vi "DCS.vi"(3 "error in":errorcluster) -> (10 "error out":errorcluster)   [LabVIEW 2012]
uses:
  Database2.0/Private/dcs points.ctl
  Database2.0/Private/dcs_spot.ctl
  <vilib>/DAQmx/read.llb/DAQmx Read (Analog 1D Wfm NChan NSamp).vi
  <vilib>/DAQmx/create/channels.llb/DAQmx Create Channel (AI-Voltage-Basic).vi
  <vilib>/DAQmx/configure/timing.llb/DAQmx Timing (Sample Clock).vi
  <vilib>/DAQmx/configure/trigger.llb/DAQmx Reference Trigger (Digital Edge).vi
  <vilib>/DAQmx/miscellaneous.llb/DAQmx Fill In Error Info.vi
  <vilib>/gmath/NumericalOptimization/Nonlinear Curve Fit LM.vi
  <vilib>/gmath/NI_Gmath.lvlib
panel:
  in  "Color bar Control":cluster{dbl, u32}[](array[cluster])
  in  "stop":bool
  in  "Tab Control":T1(tab)
  out "Intensity Graph":dbl[][](graph)
  in  "Spot Save Folder":path=path "C:/Users/Clavius/Desktop/Spot Images"
  in  "Save Spot Image":bool
  in  "Clear Spot/Track":bool
  in  "Particle Limit":i64=500 min=0 step=10
  out "Laser spot\nMove (mm)":dbl[](array[numeric])=[nan, nan] format="%#.3g"
  out "Avg. Freq. (Hz)":dbl
  in  "Orange Cursor Position":dbl[](array[numeric])=[0.0, 0.0] min=-12.0 max=12.0 step=0.1 format="%.3g"
  out "Spot Widths":dbl[](array[numeric]) format="%.6g"
  out "Countdown to\nnext track point":i32=1
  out "XY Graph":cluster{"Y":dbl[], "Y":dbl[]}[](graph)
  in  "Load old position\nto Orange Cursor":bool
  in  "Set Orange Cursor\nto current position":bool
  out "# of Particles\nin Spot":dbl
  out "Current Spot Pos":dbl[](array[numeric])=[nan, nan] format="%.3g"
  in  "# of shots to calculate spot":i32=20
  out "Spot Size over time":dbl[][](graph)
  out "Detector/trigger":waveform(dbl)[](graph)=[{"t0"=timestamp(3437998856.7399178 s since 1904-01-01), "dt"=4.999999999999997e-05, "Y"=[]}] caption="Measurement"
  out "Top to Bottom":waveform(dbl)[](graph)=[{"t0"=timestamp(0 s since 1904-01-01), "dt"=4.999999999999997e-05, "Y"=[]}, {"t0"=timestamp(0 s since 1904-01-01), "dt"=4.999999999999997e-05, "Y"=[]}, {"t0"=timestamp(0 s since 1904-01-01), "dt"=4.999999999999997e-05, "Y"=[]}, {"t0"=timestamp(0 s since 1904-01-01), "dt"=4.999999999999997e-05, "Y"=[]}] caption="Measurement"
  out "Left to Right":waveform(dbl)[](graph)=[{"t0"=timestamp(0 s since 1904-01-01), "dt"=4.999999999999997e-05, "Y"=[]}, {"t0"=timestamp(0 s since 1904-01-01), "dt"=4.999999999999997e-05, "Y"=[]}, {"t0"=timestamp(0 s since 1904-01-01), "dt"=4.999999999999997e-05, "Y"=[]}, {"t0"=timestamp(0 s since 1904-01-01), "dt"=4.999999999999997e-05, "Y"=[]}] caption="Measurement"
  out "All Signals":waveform(dbl)[](graph)=[{"t0"=timestamp(3437998856.7398734 s since 1904-01-01), "dt"=4.999999999999997e-05, "Y"=[]}, {"t0"=timestamp(3437998856.739879 s since 1904-01-01), "dt"=4.999999999999997e-05, "Y"=[]}, {"t0"=timestamp(3437998856.7398844 s since 1904-01-01), "dt"=4.999999999999997e-05, "Y"=[]}, {"t0"=timestamp(3437998856.73989 s since 1904-01-01), "dt"=4.999999999999997e-05, "Y"=[]}, {"t0"=timestamp(3437998856.739896 s since 1904-01-01), "dt"=4.999999999999997e-05, "Y"=[]}, {"t0"=timestamp(3437998856.739901 s since 1904-01-01), "dt"=4.999999999999997e-05, "Y"=[]}, {"t0"=timestamp(3437998856.739907 s since 1904-01-01), "dt"=4.999999999999997e-05, "Y"=[]}, {"t0"=timestamp(3437998856.7399125 s since 1904-01-01), "dt"=4.999999999999997e-05, "Y"=[]}, {"t0"=timestamp(3437998856.7399178 s since 1904-01-01), "dt"=4.999999999999997e-05, "Y"=[]}] caption="Measurement"
  in  "timeout":dbl=2.0 format="%0.2f"
  out "Running Errors":errorcluster
  in  "source":tag="/Dev6/PFI0"
  in  "Detector":tag="Dev6/ai8"
  in  "B2":tag="Dev6/ai4" caption="B2 /6"
  in  "B1":tag="Dev6/ai5" caption="B1 /5"
  in  "T1":tag="Dev6/ai6" caption="T1 /8"
  in  "T2":tag="Dev6/ai7" caption="T2 /7"
  in  "R2":tag="Dev6/ai3" caption="R2 /3"
  in  "R1":tag="Dev6/ai2" caption="R1 /4"
  in  "L1":tag="Dev6/ai1" caption="L1 /1"
  in  "pretrigger samples per channel":u32=120
  in  "slope":i32(ring)=10280 items=["Rising"=10280, "Falling"=10171]
  in  "Maximum Value":dbl=10.0 format="%0.2f"
  in  "Minimum Value":dbl=-10.0 format="%0.2f"
  in  "Rate":dbl=20000.0 caption="Sample Rate (Hz)" format="%0.2f"
  in  "Samples per Channel":i32=500
  in  "L2":tag="Dev6/ai0" caption="L2 /2"
  in  "Clear DCS errors":bool
  # "Channel Parameters"
  # "Timing Parameters"
  # "Trigger Parameters"
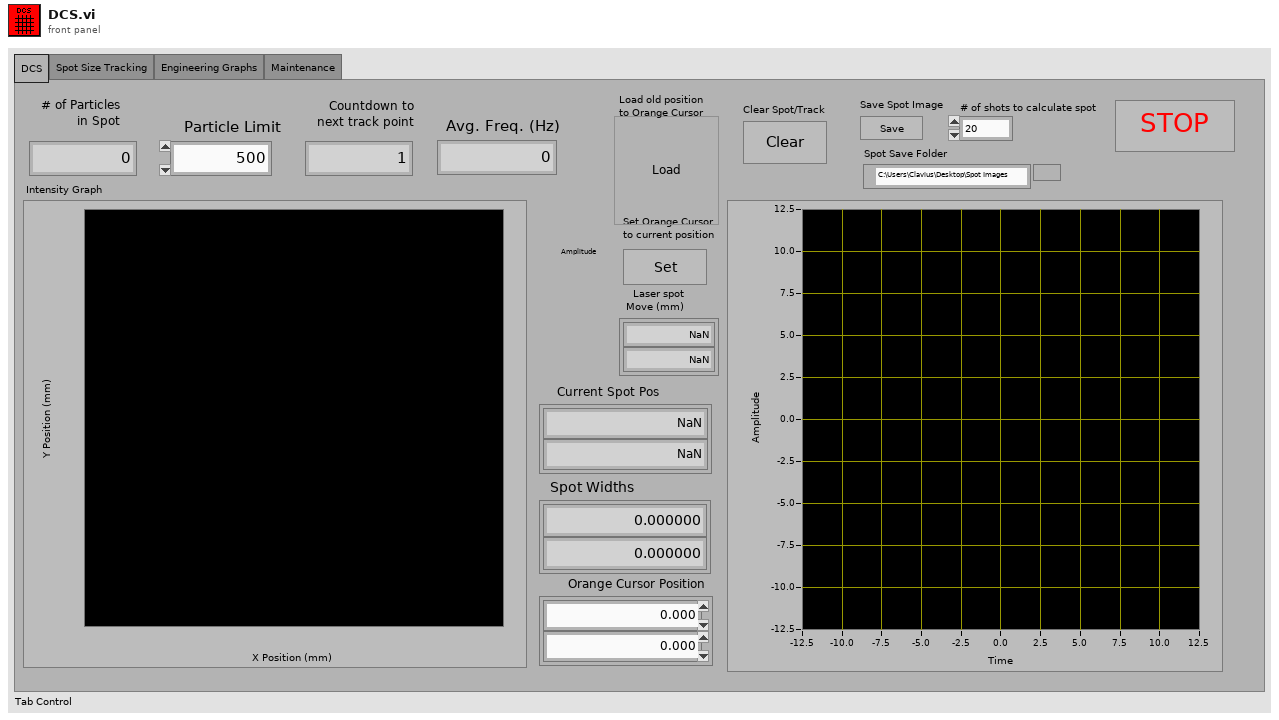
[diagram p1: front panel]
types:
  T1 = enum32{"DCS", "Spot Size Tracking", "Engineering Graphs", "Maintenance"}
  T2 = typedef "dcs_spot.ctl" = cluster{"DCS spot ID":i32, "Integer Timestamp":i64, "Spot X":dbl, "Spot Y":dbl, "Spot Width X":dbl, "Spot Width Y":dbl, "Spot Size":i32, "Experiment Settings ID":i32}
  T3 = typedef "dcs points.ctl" = cluster{"Integer Timestamp":i64, "X":dbl, "Y":dbl, "DCS spot ID":i32}
  T4 = typedef "imagedata.ctl" = cluster{"image type":i32, "image depth":i32, "image":u8[], "mask":u8[], "colors":u32[], "Rectangle":cluster{"left":i16, "top":i16, "right":i16, "bottom":i16}}
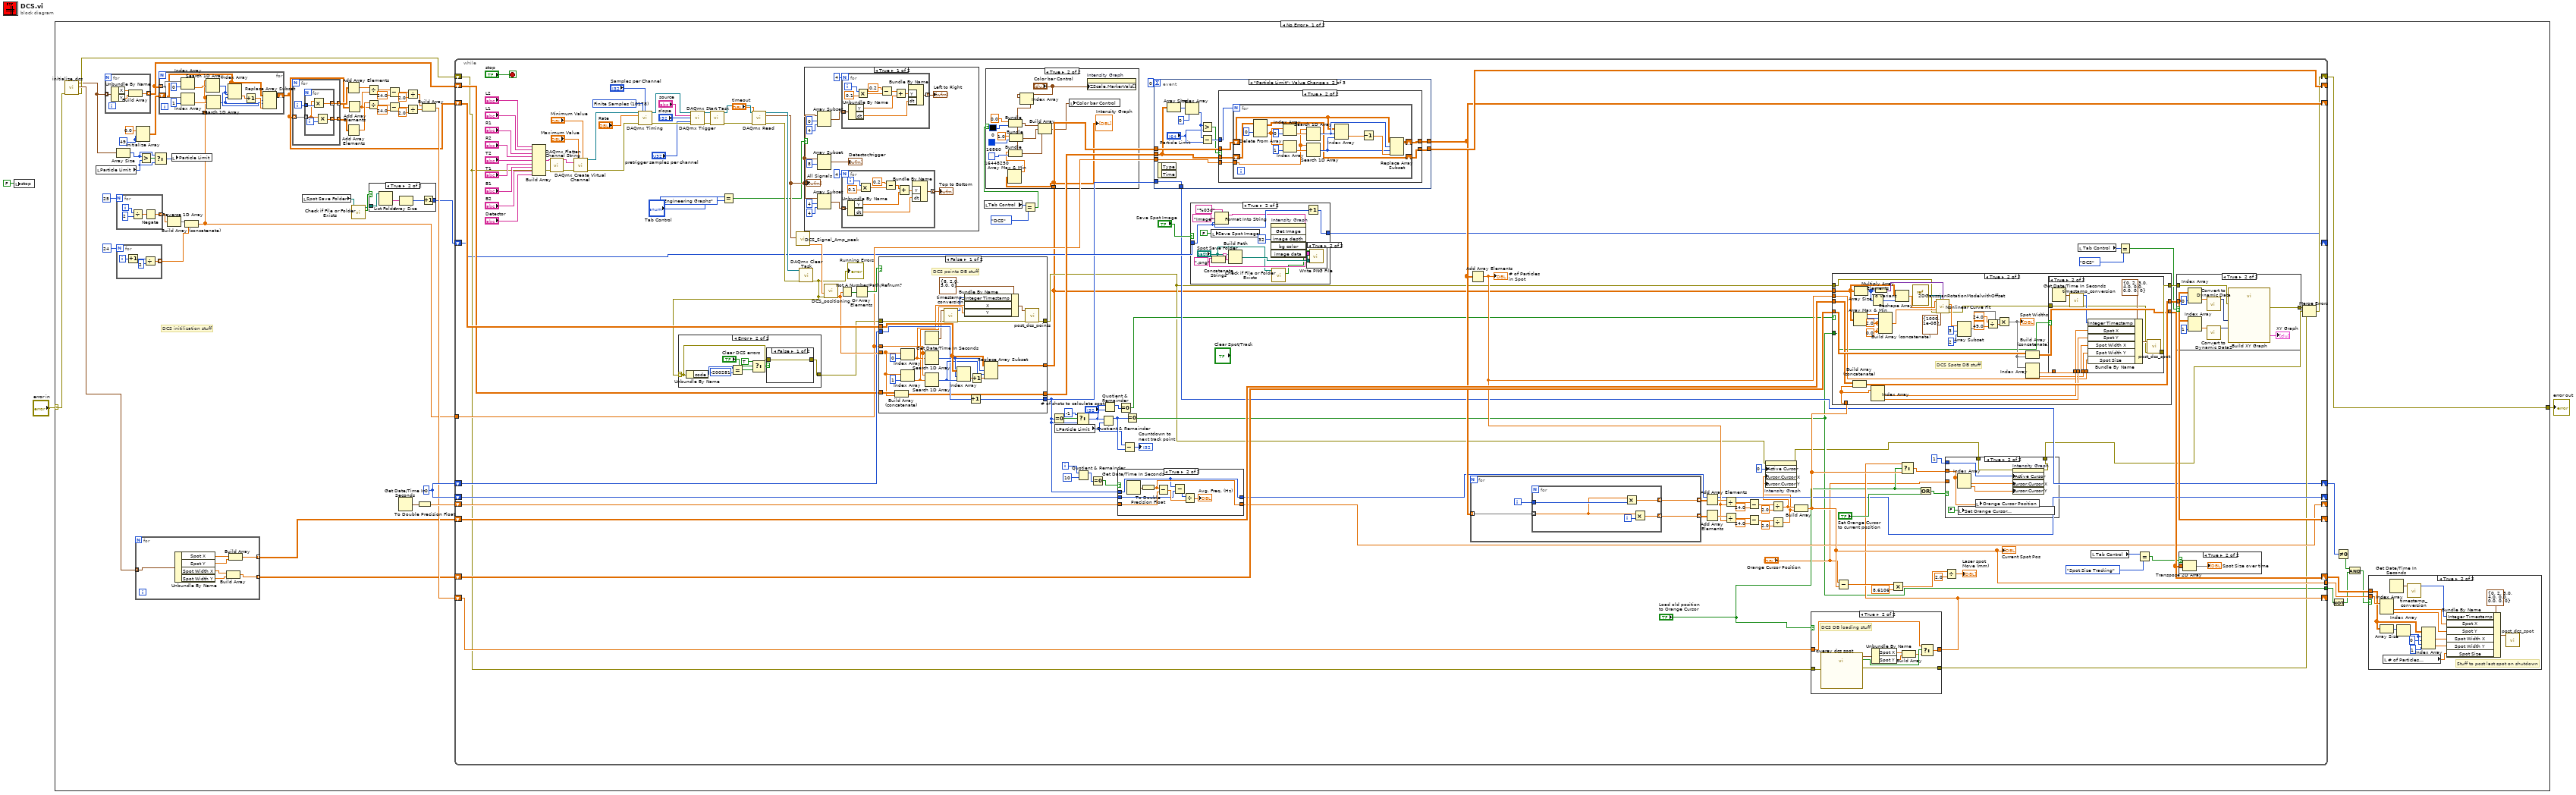
[diagram p0: block diagram]
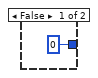
[diagram p2: hidden frame]
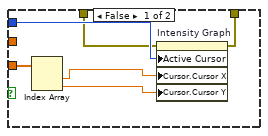
[diagram p7: hidden frame]
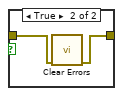
[diagram p12: hidden frame]
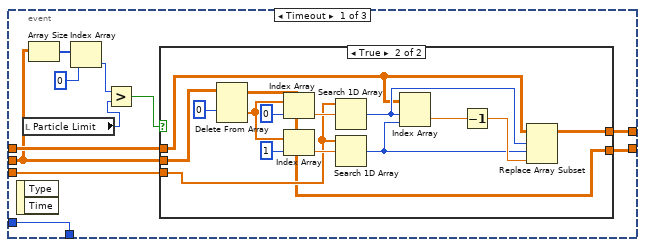
[diagram p13: hidden frame]
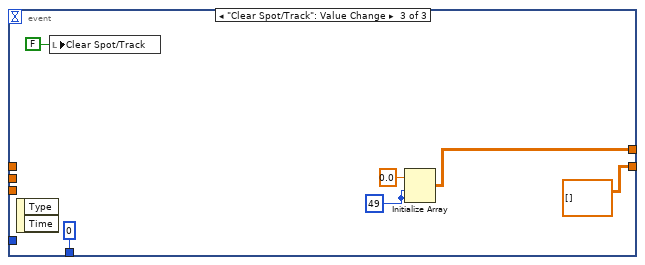
[diagram p16: hidden frame]
diagram:
  n1 = local write "stop"(FALSE ("stop")) -> ()
  n2 = case shown="No Error" "error in" {
    selector: "error in" -> [w9 w517]
    tunnel: [w8 w517] -> w2
    frame No Error {
      w30 = 49 ("dimension size")
      w33 = 0
      # "DCS initilization stuff"
      n3 = call "initialize_dcs.vi"("error in (no error)"=w9) -> ("error out"=w21:errorcluster, "Dust Spot Array"=w22:T2[], "Dust Point Array"=w14:T3[])  [unwired: 8 in]
      n4 = local read "Particle Limit"() -> (w11:i64)
      n5 = for {
        tunnel: [w81] -> w20 mode=indexing
        tunnel: w14 -> [w80] mode=indexing
        n6 = Unbundle By Name(w80) -> ("X"=w83:dbl, "Y"=w82:dbl)
        n7 = Build Array(w83, w82) -> (w81:dbl[])
      }
      n8 = for {
        N: 25 -> [_]
        tunnel: [w112] -> w53 mode=indexing
        i -> [w115]
        n9 = Divide(x=w115, y=2) -> (x/y=w113:dbl)
        n10 = Negate(x=w113) -> (-x=w112:dbl)
      }
      n11 = Array Size(array=w14) -> (size(s)=w12:i32)
      n12 = for {
        N: 24 -> [_]
        tunnel: [w109] -> w51 mode=indexing
        i -> [w111]
        n13 = Increment(x=w111) -> (x+1=w108:i32)
        n14 = Divide(x=w108, y=2) -> (x/y=w109:dbl)
      }
      n15 = for {
        tunnel: [w75] -> w25 mode=indexing
        tunnel: [w74] -> w26 mode=indexing
        tunnel: w22 -> [w73] mode=indexing
        n16 = Unbundle By Name(w73) -> ("Spot X"=w79:dbl, "Spot Y"=w78:dbl, "Spot Width X"=w77:dbl, "Spot Width Y"=w76:dbl)
        n17 = Build Array(w77, w76) -> (w75:dbl[])
        n18 = Build Array(w79, w78) -> (w74:dbl[])
      }
      n19 = Initialize Array(0.0 ("element"), w30, w30) -> (w29:dbl[][])
      n20 = Greater?(x=w12, y=w11) -> (0:w13:bool)
      n21 = Select(t=w12, s=w13, f=w11) -> (s? t:f=w10:i64)
      n22 = Reverse 1D Array(array=w53) -> (reversed array=w52:dbl[])
      n23 = local write "Particle Limit"(w10) -> ()
      n24 = Build Array (concatenate)(w52, w51) -> (w27:dbl[])
      n25 = for {
        tunnel: w20 -> [w70] mode=indexing
        tunnel: w27 -> [w61]
        shift-right: [w62] -> w19
        shift-left: w29 -> [w63]
        n26 = Index Array(array=w70, index=0) -> (element=w69:dbl)
        n27 = Index Array(array=w70, index=1) -> (element=w68:dbl)
        n28 = Search 1D Array(1D array=w61, element=w69) -> (index of element=w65:i32)  [unwired: 1 in]
        n29 = Search 1D Array(1D array=w61, element=w68) -> (index of element=w64:i32)  [unwired: 1 in]
        n30 = Index Array(array=w63, index (row)=w65, index (col)=w64) -> (element=w67:dbl)
        n31 = Increment(x=w67) -> (x+1=w66:dbl)
        n32 = Replace Array Subset(array=w63, new element=w66, index (row)=w65, index (col)=w64) -> (w62:dbl[][])
      }
      n33 = for {
        tunnel: w19 -> [w102] mode=indexing
        tunnel: [w100] -> w50 mode=indexing
        tunnel: [w99] -> w49 mode=indexing
        i -> [w101]
        n34 = for {
          tunnel: w102 -> [w104] mode=indexing
          tunnel: w101 -> [w107]
          tunnel: [w105] -> w99 mode=indexing
          tunnel: [w103] -> w100 mode=indexing
          i -> [w106]
          n35 = Multiply(x=w104, y=w107) -> (x*y=w103:dbl)
          n36 = Multiply(x=w104, y=w106) -> (x*y=w105:dbl)
        }
      }
      n37 = local read "Spot Save Folder"() -> (w6:path)
      n38 = Add Array Elements(numeric array=w50) -> (sum=w48:dbl)
      n39 = Add Array Elements(numeric array=w49) -> (sum=w47:dbl)
      n40 = Add Array Elements(numeric array=w19) -> (sum=w39:dbl)
      n41 = call <vilib>:"Check if File or Folder Exists.vi"("path"=w6) -> ("file or folder exists?"=w5:bool, "dup path"=w4:path)  [unwired: 8 in, 1 out]
      n42 = Divide(x=w48, y=w39) -> (x/y=w46:dbl)
      n43 = Divide(x=w47, y=w39) -> (x/y=w45:dbl)
      n44 = case shown="True" w5 {
        tunnel: [0 w58] -> w7
        tunnel: w4 -> [_ w57]
        frame False {
        }
        frame True {
          n45 = List Folder(path=w57) -> (filenames=w60:string[])  [unwired: 3 in, 3 out]
          n46 = Array Size(array=w60) -> (size(s)=w59:i32)
          n47 = Increment(x=w59) -> (x+1=w58:i32)
        }
      }
      n48 = Subtract(x=w46, y=24.0) -> (x-y=w37:dbl)
      n49 = Subtract(x=w45, y=24.0) -> (x-y=w43:dbl)
      n50 = Get Date/Time In Seconds() -> (seconds since 1Jan1904=w35:timestamp)
      n51 = Divide(x=w37, y=2.0) -> (x/y=w36:dbl)
      n52 = Divide(x=w43, y=2.0) -> (x/y=w40:dbl)
      n53 = To Double Precision Float(number=w35) -> (double precision float=w34:dbl)
      n54 = Build Array(w36, w40) -> (w28:dbl[])
      n55 = while {
        shift-right: [w183] -> _
        shift-left: w20 -> [w185]
        shift-right: [w168] -> _
        shift-left: w19 -> [w208]
        tunnel: w27 -> [w159]
        shift-right: [w167] -> _
        shift-left: w28 -> [w196]
        tunnel: [w182] -> w32
        shift-right: [w158] -> w8
        shift-left: w21 -> [w152]
        shift-right: [w180] -> _
        shift-left: w26 -> [w172]
        shift-right: [w146] -> w18
        shift-left: w33 -> [w186]
        shift-right: [w181] -> w23
        shift-left: w25 -> [w184]
        shift-right: [w165] -> _
        shift-left: w34 -> [w179]
        shift-right: [w164] -> _
        shift-left: w33 -> [w166]
        tunnel: [w142] -> w24
        shift-right: [w148] -> _
        shift-left: w7 -> [w149]
        i -> [w125]
        stop <- "stop" stop-if-true
        w233 = 10178 items=["Finite Samples"=10178, "Continuous Samples"=10123] ("sample mode")
        n56 = Build Array("L2", "L1", "R1", "R2", "T2", "T1", "B1", "B2", "Detector") -> (w223:tag[])
        n57 = call <vilib>:"DAQmx Flatten Channel String.vi"("names in"=w223, "error in"=w152) -> ("names out"=w221:string, "error out"=w222:errorcluster)  [unwired: 12 in]
        n58 = call-poly <vilib>:"DAQmx Create Virtual Channel.vi"("maximum value"="Maximum Value", "minimum value"="Minimum Value", "physical channels"=w221, "error in"=w222) -> ("task out"=w236:refnum<k21>, "error out"=w240:errorcluster)  [unwired: 10 in]
        n59 = call-poly <vilib>:"DAQmx Timing.vi"("task/channels in"=w236, "sample mode"=w233, "samples per channel"="Samples per Channel", "rate"="Rate", "error in"=w240) -> ("task out"=w231:refnum<k21>, "error out"=w230:errorcluster)  [unwired: 9 in]
        n60 = call-poly <vilib>:"DAQmx Trigger.vi"("task/channels in"=w231, "source"="source", "edge"="slope", "error in"=w230, "pretrigger samples per channel"="pretrigger samples per channel") -> ("task out"=w228:refnum<k21>, "error out"=w229:errorcluster)  [unwired: 9 in]
        n61 = call <vilib>:"DAQmx Start Task.vi"("task/channels in"=w228, "error in"=w229) -> ("task out"=w235:refnum<k21>, "error out"=w239:errorcluster)  [unwired: 12 in]
        n62 = Equal?(x="Tab Control", y=T1."Engineering Graphs") -> (x = y?=w136:bool)
        n63 = call-poly <vilib>:"DAQmx Read.vi"("task/channels in"=w235, "timeout"="timeout", "error in"=w239) -> ("task out"=w234:refnum<k21>, "data"=w209:waveform(dbl)[], "error out"=w232:errorcluster)  [unwired: 10 in]
        n64 = call "DCS_Signal_Amp_peak.vi"("data"=w209) -> ("Data"=w210:dbl[])  [unwired: 10 in]
        n65 = call <vilib>:"DAQmx Clear Task.vi"("task in"=w234, "error in"=w232) -> ("error out"=w157:errorcluster)  [unwired: 13 in]
        "Running Errors" <- w157
        n66 = case shown="Error" w157 {
          selector: w157 -> [w329 w335]
          tunnel: [w329 w334] -> w156
          frame No Error {
          }
          frame Error {
            n67 = Unbundle By Name(w335) -> ("code"=w337:i32)
            n68 = Equal?(x=w337, y=-200281) -> (x = y?=w333:bool)
            n69 = Select(t=TRUE, s="Clear DCS errors", f=w333) -> (s? t:f=w332:bool)
            n70 = case shown="False" w332 {
              tunnel: w335 -> [w338 w340]
              tunnel: [w338 w339] -> w334
              frame False {
              }
              frame True {
                n71 = call <vilib>:"Clear Errors.vi"("error in (no error)"=w340) -> ("error out"=w339:errorcluster)  [unwired: 6 in]
              }
            }
          }
        }
        n72 = case shown="True" w136 {
          tunnel: w209 -> [w282 _]
          frame True {
            n73 = Array Subset(array=w282, index=0, length=4) -> (w284:waveform(dbl)[])
            n74 = Array Subset(array=w282, index=8) -> (→"Detector/trigger":waveform(dbl)[])  [unwired: 1 in]
            n75 = Array Subset(array=w282, index=4, length=4) -> (w283:waveform(dbl)[])
            n76 = for {
              N: 4 -> [_]
              tunnel: [w295] -> w291 mode=indexing
              tunnel: w284 -> [w294] mode=indexing
              i -> [w299]
              n77 = Unbundle By Name(w294) -> ("Y"=w301:dbl[], "dt"=w302:dbl)
              n78 = Multiply(x=w299, y=0.1) -> (x*y=w298:dbl)
              n79 = Subtract(x=0.2, y=w298) -> (x-y=w296:dbl)
              n80 = Add(x=w296, y=w301) -> (x+y=w293:dbl[])
              n81 = Bundle By Name("Y"=w293, "dt"=w302) -> (w295:waveform(dbl))  [unwired: 1 in]
            }
            "Left to Right" <- w291
            n82 = for {
              N: 4 -> [_]
              tunnel: [w305] -> w289 mode=indexing
              tunnel: w283 -> [w304] mode=indexing
              i -> [w309]
              n83 = Unbundle By Name(w304) -> ("Y"=w311:dbl[], "dt"=w312:dbl)
              n84 = Multiply(x=w309, y=0.1) -> (x*y=w308:dbl)
              n85 = Subtract(x=0.2, y=w308) -> (x-y=w306:dbl)
              n86 = Add(x=w306, y=w311) -> (x+y=w303:dbl[])
              n87 = Bundle By Name("Y"=w303, "dt"=w312) -> (w305:waveform(dbl))  [unwired: 1 in]
            }
            "Top to Bottom" <- w289
            "All Signals" <- w282
          }
          frame False {
          }
        }
        n88 = call "DCS_positioning.vi"("error in (no error)"=w157, "Data"=w210) -> ("X-Y position"=w193:dbl[])  [unwired: 9 in]
        n89 = Not A Number/Path/Refnum?(number/path/refnum=w193) -> (NaN/Path/Refnum?=w207:bool[])
        n90 = Or Array Elements(Boolean array=w207) -> (logical OR=w192:bool)
        n91 = case shown="False" w192 {
          tunnel: w208 -> [w510 w516]
          tunnel: [w505 w516] -> w126
          tunnel: w159 -> [w504 _]
          tunnel: w193 -> [w500 _]
          tunnel: w186 -> [w503 w515]
          tunnel: [w502 w515] -> w147
          tunnel: w185 -> [w501 w514]
          tunnel: [w499 w514] -> w162
          tunnel: w156 -> [w495 w513]
          tunnel: [w494 w513] -> w131
          frame False {
            # "DCS points DB stuff"
            n92 = Build Array (concatenate)(w501, w500) -> (w499:dbl[][])
            n93 = Index Array(array=w500, index=0) -> (element=w498:dbl)
            n94 = Index Array(array=w500, index=1) -> (element=w497:dbl)
            n95 = Get Date/Time In Seconds() -> (seconds since 1Jan1904=w496:timestamp)
            n96 = Search 1D Array(1D array=w504, element=w498) -> (index of element=w509:i32)  [unwired: 1 in]
            n97 = Search 1D Array(1D array=w504, element=w497) -> (index of element=w508:i32)  [unwired: 1 in]
            n98 = call "timestamp_conversion.vi"("error in (no error)"=w495, "Time Stamp"=w496) -> ("error out"=w490:errorcluster, "Integer Time"=w493:i64)  [unwired: 7 in]
            n99 = Index Array(array=w510, index (row)=w509, index (col)=w508) -> (element=w507:dbl)
            n100 = Bundle By Name(cluster=T3 {"Integer Timestamp"=8, "X"=2.0, "Y"=3.0, "DCS spot ID"=0} ("DCS points"), "Integer Timestamp"=w493, "X"=w498, "Y"=w497) -> (w492:T3)
            n101 = Increment(x=w503) -> (x+1=w502:i32)
            n102 = Increment(x=w507) -> (x+1=w506:dbl)
            n103 = Replace Array Subset(array=w510, new element=w506, index (row)=w509, index (col)=w508) -> (w505:dbl[][])
            n104 = call "post_dcs_points.vi"("error in (no error)"=w490, "DCS points"=w492) -> ("error out"=w494:errorcluster)  [unwired: 8 in, 1 out]
          }
          frame True {
          }
        }
        n105 = local read "Tab Control"() -> (w118:T1)
        n106 = Equal?(x=w118, y=T1."DCS") -> (x = y?=w116:bool)
        n107 = case shown="True" w116 {
          tunnel: w126 -> [_ w243]
          frame False {
          }
          frame True {
            n108 = Array Max & Min(array=w243) -> (max value=w242:dbl)  [unwired: 3 out]
            n109 = Index Array(array="Color bar Control") -> (element=w251:cluster{dbl, u32})  [unwired: 1 in]
            n110 = Bundle(cluster=w251, 0.0, u32 0) -> (w252:cluster{dbl, u32})
            n111 = Bundle(cluster=w251, w242, u32 16448250) -> (w249:cluster{dbl, u32})
            n112 = Bundle(cluster=w251, 1.0, u32 16860) -> (w250:cluster{dbl, u32})
            n113 = Build Array(w252, w250, w249) -> (w241:cluster{dbl, u32}[])
            n114 = local write "Color bar Control"(w241) -> ()
            n115 = property on="Intensity Graph" class="IntGraph (strict)"("ZScale.MarkerVals[]"="Color bar Control") -> ()  [unwired: 2 in, 2 out]
            "Intensity Graph" <- w243
          }
        }
        n116 = Equal To 0?(x=w147) -> (x = 0?=w190:bool)
        n117 = local read "Particle Limit"() -> (w155:i64)
        n118 = Select(t=-1, s=w190, f=w147) -> (s? t:f=w154:i32)
        n119 = Quotient & Remainder(x=w125, y=10) -> (x-y*floor(x/y)=w178:i32)  [unwired: 1 out]
        n120 = Equal To 0?(x=w178) -> (x = 0?=w123:bool)
        n121 = Quotient & Remainder(x=w154, y=w155) -> (x-y*floor(x/y)=w188:i64)  [unwired: 1 out]
        n122 = Quotient & Remainder(x=w154, y="# of shots to calculate spot") -> (x-y*floor(x/y)=w153:i32)  [unwired: 1 out]
        n123 = case shown="True" w123 {
          tunnel: w179 -> [w411 w418]
          tunnel: [w411 w415] -> w165
          tunnel: [w410 w414] -> w164
          tunnel: w166 -> [w410 w413]
          tunnel: w147 -> [_ w414]
          frame False {
          }
          frame True {
            n124 = Get Date/Time In Seconds() -> (seconds since 1Jan1904=w419:timestamp)
            n125 = To Double Precision Float(number=w419) -> (double precision float=w415:dbl)
            n126 = Subtract(x=w415, y=w418) -> (x-y=w417:dbl)
            n127 = Subtract(x=w414, y=w413) -> (x-y=w412:i32)
            n128 = Divide(x=w412, y=w417) -> (x/y=→"Avg. Freq. (Hz)":dbl)
          }
        }
        n129 = Equal To 0?(x=w153) -> (x = 0?=w141:bool)
        n130 = Subtract(x=w155, y=w188) -> (x-y=→"Countdown to\nnext track point":i64)
        n131 = Equal To 0?(x=w188) -> (x = 0?=w142:bool)
        n132 = event shown="[1] \"Particle Limit\": Value Change" {
          selector: _ -> [_ _ _]
          dyn-events: _ -> [_ _ _]
          timeout: 0 -> [_ _ _]
          tunnel: w159 -> [w351 w379 _]
          tunnel: w126 -> [w350 w380 _]
          tunnel: [w349 w378 w406] -> w168
          tunnel: w162 -> [w343 w370 _]
          tunnel: [w348 w377 dbl[][] []] -> w183
          tunnel: w147 -> [w341 w369 _]
          tunnel: [w341 w369 0] -> w146
          event Timeout {
            n133 = event-data() -> ()  [unwired: 1 in, 2 out]
            n134 = local read "Particle Limit"() -> (w344:i64)
            n135 = Array Size(array=w343) -> (size(s)=w347:i32[])
            n136 = Index Array(array=w347, index=0) -> (element=w345:i32)
            n137 = Greater?(x=w345, y=w344) -> (0:w342:bool)
            n138 = case shown="True" w342 {
              tunnel: w351 -> [_ w364]
              tunnel: w350 -> [w353 w359]
              tunnel: [w353 w358] -> w349
              tunnel: w343 -> [w352 w357]
              tunnel: [w352 w354] -> w348
              frame False {
              }
              frame True {
                n139 = Delete From Array(array=w357, index (row)=0) -> (deleted portion=w355:dbl[], array with subset deleted=w354:dbl[][])  [unwired: 2 in]
                n140 = Index Array(array=w355, index=0) -> (element=w365:dbl)
                n141 = Index Array(array=w355, index=1) -> (element=w366:dbl)
                n142 = Search 1D Array(1D array=w364, element=w365) -> (index of element=w360:i32)  [unwired: 1 in]
                n143 = Search 1D Array(1D array=w364, element=w366) -> (index of element=w361:i32)  [unwired: 1 in]
                n144 = Index Array(array=w359, index (row)=w360, index (col)=w361) -> (element=w363:dbl)
                n145 = Decrement(x=w363) -> (x-1=w362:dbl)
                n146 = Replace Array Subset(array=w359, new element=w362, index (row)=w360, index (col)=w361) -> (w358:dbl[][])
              }
            }
          }
          event "Particle Limit": Value Change {
            n147 = event-data() -> ()  [unwired: 1 in, 2 out]
            n148 = Array Size(array=w370) -> (size(s)=w376:i32[])
            n149 = Index Array(array=w376, index=0) -> (element=w374:i32)
            n150 = Greater?(x=w374, y="Particle Limit") -> (0:w371:bool)
            n151 = Subtract(x=w374, y="Particle Limit") -> (x-y=w372:i64)
            n152 = case shown="True" w371 {
              tunnel: w380 -> [w382 w386]
              tunnel: w370 -> [w381 w388]
              tunnel: w379 -> [_ w387]
              tunnel: [w381 w385] -> w377
              tunnel: [w382 w384] -> w378
              tunnel: w372 -> [_ w383]
              frame False {
              }
              frame True {
                n153 = for {
                  N: w383 -> [_]
                  tunnel: w387 -> [w393]
                  shift-right: [w389] -> w384
                  shift-left: w386 -> [w392]
                  shift-right: [w390] -> w385
                  shift-left: w388 -> [w394]
                  n154 = Delete From Array(array=w394, index (row)=0) -> (deleted portion=w391:dbl[], array with subset deleted=w390:dbl[][])  [unwired: 2 in]
                  n155 = Index Array(array=w391, index=0) -> (element=w400:dbl)
                  n156 = Index Array(array=w391, index=1) -> (element=w401:dbl)
                  n157 = Search 1D Array(1D array=w393, element=w400) -> (index of element=w396:i32)  [unwired: 1 in]
                  n158 = Search 1D Array(1D array=w393, element=w401) -> (index of element=w397:i32)  [unwired: 1 in]
                  n159 = Index Array(array=w392, index (row)=w396, index (col)=w397) -> (element=w399:dbl)
                  n160 = Decrement(x=w399) -> (x-1=w398:dbl)
                  n161 = Replace Array Subset(array=w392, new element=w398, index (row)=w396, index (col)=w397) -> (w389:dbl[][])
                }
              }
            }
          }
          event "Clear Spot/Track": Value Change {
            w407 = 49 ("dimension size")
            n162 = event-data() -> ()  [unwired: 1 in, 2 out]
            n163 = local write "Clear Spot/Track"(FALSE ("Clear Spot/Track")) -> ()
            n164 = Initialize Array(0.0 ("element"), w407, w407) -> (w406:dbl[][])
          }
        }
        n165 = case shown="True" "Save Spot Image" {
          tunnel: w149 -> [w313 w323]
          tunnel: [w313 w322] -> w148
          frame False {
          }
          frame True {
            n166 = local write "Save Spot Image"(FALSE ("Save Spot Image")) -> ()
            n167 = Format Into String(format string="%03d", initial string="Image", w323) -> (resulting string=w319:string)  [unwired: 1 in, 1 out]
            n168 = Concatenate Strings(w319, ".png" ("string")) -> (w320:string)
            n169 = Build Path(base path="Spot Save Folder", name or relative path=w320) -> (appended path=w321:path)
            n170 = invoke on="Intensity Graph" class="IntGraph (strict)" method="Get Image"("image depth"=32 ("Image Depth")) -> ("image data"=w317:T4)  [unwired: 5 in, 5 out]
            n171 = call <vilib>:"Check if File or Folder Exists.vi"("path"="Spot Save Folder") -> ("file or folder exists?"=w314:bool)  [unwired: 8 in, 2 out]
            n172 = Increment(x=w323) -> (x+1=w322:i32)
            n173 = case shown="True" w314 {
              tunnel: w321 -> [_ w328]
              tunnel: w317 -> [_ w327]
              frame False {
              }
              frame True {
                n174 = call <vilib>:"Write PNG File.vi"("image data"=w327, "path to PNG file"=w328) -> ()  [unwired: 8 in, 2 out]
              }
            }
          }
        }
        n175 = for {
          tunnel: w168 -> [w484] mode=indexing
          tunnel: [w482] -> w206 mode=indexing
          tunnel: [w481] -> w205 mode=indexing
          i -> [w483]
          n176 = for {
            tunnel: w484 -> [w486] mode=indexing
            tunnel: w483 -> [w489]
            tunnel: [w487] -> w481 mode=indexing
            tunnel: [w485] -> w482 mode=indexing
            i -> [w488]
            n177 = Multiply(x=w486, y=w489) -> (x*y=w485:dbl)
            n178 = Multiply(x=w486, y=w488) -> (x*y=w487:dbl)
          }
        }
        n179 = Add Array Elements(numeric array=w168) -> (sum=w171:dbl)
        "# of Particles\nin Spot" <- w171
        n180 = Add Array Elements(numeric array=w206) -> (sum=w204:dbl)
        n181 = Add Array Elements(numeric array=w205) -> (sum=w203:dbl)
        n182 = Divide(x=w204, y=w171) -> (x/y=w202:dbl)
        n183 = Divide(x=w203, y=w171) -> (x/y=w201:dbl)
        n184 = Subtract(x=w202, y=24.0) -> (x-y=w195:dbl)
        n185 = Subtract(x=w201, y=24.0) -> (x-y=w199:dbl)
        n186 = Divide(x=w195, y=2.0) -> (x/y=w129:dbl)
        n187 = Divide(x=w199, y=2.0) -> (x/y=w128:dbl)
        n188 = property on="Intensity Graph" class="IntGraph (strict)"(error in=w131, "Active Cursor"=u32 0, "Cursor.Cursor X"=w129, "Cursor.Cursor Y"=w128) -> (error out=w130:errorcluster)  [unwired: 1 in, 1 out]
        n189 = Build Array(w129, w128) -> (w182:dbl[])
        "Current Spot Pos" <- w182
        n190 = case shown="True" "Load old position\nto Orange Cursor" {
          tunnel: [w471 w476] -> w167
          tunnel: w196 -> [w471 w473]
          tunnel: w152 -> [w470 w478]
          tunnel: [w470 w477] -> w163
          frame False {
          }
          frame True {
            # "DCS DB loading stuff"
            n191 = call "querey dcs spot.vi"("error in (no error)"=w478) -> ("Spot"=w472:T2, "Cancel loading"=w475:bool, "error out"=w477:errorcluster)  [unwired: 15 in, 1 out]
            n192 = Unbundle By Name(w472) -> ("Spot X"=w480:dbl, "Spot Y"=w479:dbl)
            n193 = Build Array(w480, w479) -> (w474:dbl[])
            n194 = Select(t=w473, s=w475, f=w474) -> (s? t:f=w476:dbl[])
          }
        }
        n195 = case shown="True" w141 {
          tunnel: w184 -> [w422 w456]
          tunnel: [w422 w424] -> w181
          tunnel: w126 -> [_ w437]
          tunnel: w172 -> [w421 w436]
          tunnel: w182 -> [_ w434]
          tunnel: [w421 w435] -> w180
          tunnel: w171 -> [_ w428]
          tunnel: [w420 w427] -> w170
          tunnel: w131 -> [w420 w425]
          tunnel: w142 -> [_ w423]
          frame False {
          }
          frame True {
            w447 = sgl 0.0 ("element")
            w448 = sgl 2.0 ("element")
            # "DCS Spots DB stuff"
            n196 = Build Array (concatenate)(w436, w434) -> (w435:dbl[][])
            n197 = Array Max & Min(array=w437) -> (max value=w450:dbl, max index (indices)=w449:i32[])  [unwired: 2 out]
            n198 = Array Size(array=w437) -> (size(s)=w453:i32[])
            n199 = Index Array(array=w434) -> (element #1=w433:dbl, element #2=w432:dbl)  [unwired: 2 in]
            n200 = Multiply Array Elements(1:w453) -> (0:w454:i32)
            n201 = To Variant(anything=w453) -> (Variant=w452:variant)
            n202 = Build Array (concatenate)(w450, w449, w448, w448, w447, w447) -> (w446:dbl[])
            n203 = Reshape Array(w437, w454) -> (w451:dbl[])
            n204 = vi-ref "2DGaussianRotationModelwithOffset.vi"() -> (w455:refnum<vi>)
            n205 = call-poly <vilib>:"Nonlinear Curve Fit.vi"("Y"=w451, "f(x,a)"=w455, "data"=w452, "initial parameters"=w446, "error in (no error)"=w425, "termination"=cluster{"max iteration":i32, "tolerance":dbl} {"max iteration"=1000, "tolerance"=1e-08}) -> ("best fit parameters"=w439:dbl[], "error out"=w426:errorcluster)  [unwired: 4 in, 4 out]
            n206 = Array Subset(array=w439, index=3, length=2) -> (w442:dbl[])
            n207 = Divide(x=24.0 ("y"), y=49.0) -> (x/y=w438:dbl)
            n208 = Multiply(x=w442, y=w438) -> (x*y=w431:dbl[])
            "Spot Widths" <- w431
            n209 = Build Array (concatenate)(w456, w431) -> (w424:dbl[][])
            n210 = Index Array(array=w431) -> (element #1=w430:dbl, element #2=w429:dbl)  [unwired: 2 in]
            n211 = case shown="True" w423 {
              tunnel: w433 -> [_ w465]
              tunnel: w432 -> [_ w464]
              tunnel: w430 -> [_ w463]
              tunnel: w429 -> [_ w462]
              tunnel: w428 -> [_ w461]
              tunnel: [w457 w459] -> w427
              tunnel: w426 -> [w457 w458]
              frame False {
              }
              frame True {
                n212 = Get Date/Time In Seconds() -> (seconds since 1Jan1904=w466:timestamp)
                n213 = call "timestamp_conversion.vi"("error in (no error)"=w458, "Time Stamp"=w466) -> ("error out"=w460:errorcluster, "Integer Time"=w469:i64)  [unwired: 7 in]
                n214 = Bundle By Name(cluster=T2 {"DCS spot ID"=0, "Integer Timestamp"=2, "Spot X"=3.0, "Spot Y"=4.0, "Spot Width X"=0.0, "Spot Width Y"=0.0, "Spot Size"=0, "Experiment Settings ID"=0} ("dcs_spot"), "Integer Timestamp"=w469, "Spot X"=w465, "Spot Y"=w464, "Spot Width X"=w463, "Spot Width Y"=w462, "Spot Size"=w461) -> (w468:T2)
                n215 = call "post_dcs_spot.vi"("error in (no error)"=w460, "dcs_spot"=w468) -> ("error out"=w459:errorcluster)  [unwired: 8 in, 1 out]
              }
            }
          }
        }
        n216 = Subtract(x="Orange Cursor Position", y=w182) -> (x-y=w177:dbl[])
        n217 = Multiply(x=w177, y=8.6106) -> (x*y=w175:dbl[])
        n218 = Select(t=w167, s="Load old position\nto Orange Cursor", f=w182) -> (s? t:f=w135:dbl[])
        n219 = Or(x="Load old position\nto Orange Cursor", y="Set Orange Cursor\nto current position") -> (x .or. y?=w134:bool)
        n220 = Divide(x=w175, y=2.0) -> (x/y=→"Laser spot\nMove (mm)":dbl[])
        n221 = case shown="True" w134 {
          tunnel: "Orange Cursor Position" -> [w272 _]
          tunnel: w135 -> [_ w279]
          tunnel: 1 -> [w269 w277]
          tunnel: w130 -> [w268 w274]
          tunnel: [w267 w273] -> w132
          frame False {
            n222 = Index Array(array=w272) -> (element #1=w271:dbl, element #2=w270:dbl)  [unwired: 2 in]
            n223 = property on="Intensity Graph" class="IntGraph (strict)"(error in=w268, "Active Cursor"=w269, "Cursor.Cursor X"=w271, "Cursor.Cursor Y"=w270) -> (error out=w267:errorcluster)  [unwired: 1 in, 1 out]
          }
          frame True {
            n224 = Index Array(array=w279) -> (element #1=w276:dbl, element #2=w275:dbl)  [unwired: 2 in]
            n225 = local write "Set Orange Cursor\nto current position"(FALSE ("Set Orange Cursor\nto current position")) -> ()
            n226 = local write "Orange Cursor Position"(w279) -> ()
            n227 = property on="Intensity Graph" class="IntGraph (strict)"(error in=w274, "Active Cursor"=w277, "Cursor.Cursor X"=w276, "Cursor.Cursor Y"=w275) -> (error out=w273:errorcluster)  [unwired: 1 in, 1 out]
          }
        }
        n228 = local read "Tab Control"() -> (w120:T1)
        n229 = local read "Tab Control"() -> (w140:T1)
        n230 = Equal?(x=w120, y=T1."DCS") -> (x = y?=w119:bool)
        n231 = Equal?(x=w140, y=T1."Spot Size Tracking") -> (x = y?=w122:bool)
        n232 = case shown="True" w119 {
          tunnel: w180 -> [_ w264]
          tunnel: w170 -> [w254 w263]
          tunnel: [w254 w262] -> w169
          frame False {
          }
          frame True {
            n233 = Index Array(array=w264, index (col)=0 ("disabled index (col)")) -> (element=w258:dbl[])  [unwired: 1 in]
            n234 = Index Array(array=w264, index (col)=1 ("disabled index (col)")) -> (element=w256:dbl[])  [unwired: 1 in]
            n235 = call "Convert to Dynamic Data"("Array"=w258) -> ("Dynamic Data Type"=w257:dynamicdata)  [unwired: 3 in]
            n236 = call "Convert to Dynamic Data2"("Array"=w256) -> ("Dynamic Data Type"=w255:dynamicdata)  [unwired: 3 in]
            n237 = call "Build XY Graph"("error in (no error)"=w263, "Y Input"=w255, "X Input"=w257) -> ("error out"=w262:errorcluster, "XY Graph"=→"XY Graph":cluster{"Y":dbl[], "Y":dbl[]}[])  [unwired: 2 in, 5 out]
          }
        }
        n238 = case shown="True" w122 {
          tunnel: w181 -> [_ w266]
          frame False {
          }
          frame True {
            n239 = Transpose 2D Array(2D array=w266) -> (transposed array=→"Spot Size over time":dbl[][])
          }
        }
        n240 = Merge Errors(w169, w132, w163) -> (w158:errorcluster)
      }
      n241 = Not(x=w24) -> (.not. x?=w17:bool)
      n242 = Not Equal To 0?(x=w18) -> (x != 0?=w15:bool)
      n243 = And(x=w15, y=w17) -> (x .and. y?=w16:bool)
      n244 = case shown="True" w16 {
        tunnel: w32 -> [_ w94]
        tunnel: w23 -> [_ w90]
        frame False {
        }
        frame True {
          # "Stuff to post last spot on shutdown"
          n245 = Index Array(array=w94) -> (element #1=w93:dbl, element #2=w92:dbl)  [unwired: 2 in]
          n246 = Array Size(array=w90) -> (size(s)=w91:i32[])
          n247 = local read "# of Particles\nin Spot"() -> (w84:dbl)
          n248 = Get Date/Time In Seconds() -> (seconds since 1Jan1904=w98:timestamp)
          n249 = Index Array(array=w91) -> (element=w89:i32)  [unwired: 1 in]
          n250 = call "timestamp_conversion.vi"("Time Stamp"=w98) -> ("Integer Time"=w97:i64)  [unwired: 8 in, 1 out]
          n251 = Index Array(array=w90, index (row) #1=w89, index (col) #1=0 ("disabled index (col)"), index (row) #2=w89, index (col) #2=1 ("disabled index (col)")) -> (element #1=w88:dbl, element #2=w85:dbl)
          n252 = Bundle By Name(cluster=T2 {"DCS spot ID"=0, "Integer Timestamp"=2, "Spot X"=3.0, "Spot Y"=4.0, "Spot Width X"=0.0, "Spot Width Y"=0.0, "Spot Size"=0, "Experiment Settings ID"=0} ("dcs_spot"), "Integer Timestamp"=w97, "Spot X"=w93, "Spot Y"=w92, "Spot Width X"=w88, "Spot Width Y"=w85, "Spot Size"=w84) -> (w95:T2)
          n253 = call "post_dcs_spot.vi"("dcs_spot"=w95) -> ()  [unwired: 9 in, 2 out]
        }
      }
    }
    frame Error {
    }
  }
  "error out" <- w2
